vi "Waveform Axis Parameters.vi"(7 "Image Acquisition Parameters":T2={"Scan Type"=enum."Sample Scanning", "Scan Mode"=enum."XY", "Fast Axis Frequency (Hz)"=100.0, "Image Format"=128, "Line Accumulations"=1, "Frames Per Capture"=1, "Frames Accumulations"=1, "Image Dimension (um)"=[], "Number of Z Steps"=1, "Z Steps Size (um)"=1.0, "Pixel Size (nm)"=[], "Customized Image Format"=[]} {"Z Steps Size (um)" min=0.0; "Number of Z Steps" min=1; "Frames Accumulations" min=1; "Frames Per Capture" min=1; "Line Accumulations" min=1; "Image Format" items=["64 x 64"=64, "128 x 128"=128, "256 x 256"=256, "512 x 512"=512, "1024 x 1024"=1024, "2048 x 2048"=2048, "Customized..."=0]}) -> (8 "Scan Parameters":T1)   [LabVIEW 2014]
uses:
  Type Defs/Image Acquisition Parameters.ctl
  Scan Parameters.ctl
panel:
  # "Length"
  # "Height"
  # "XY"
  # "Z"
  # "Length"
  # "Height"
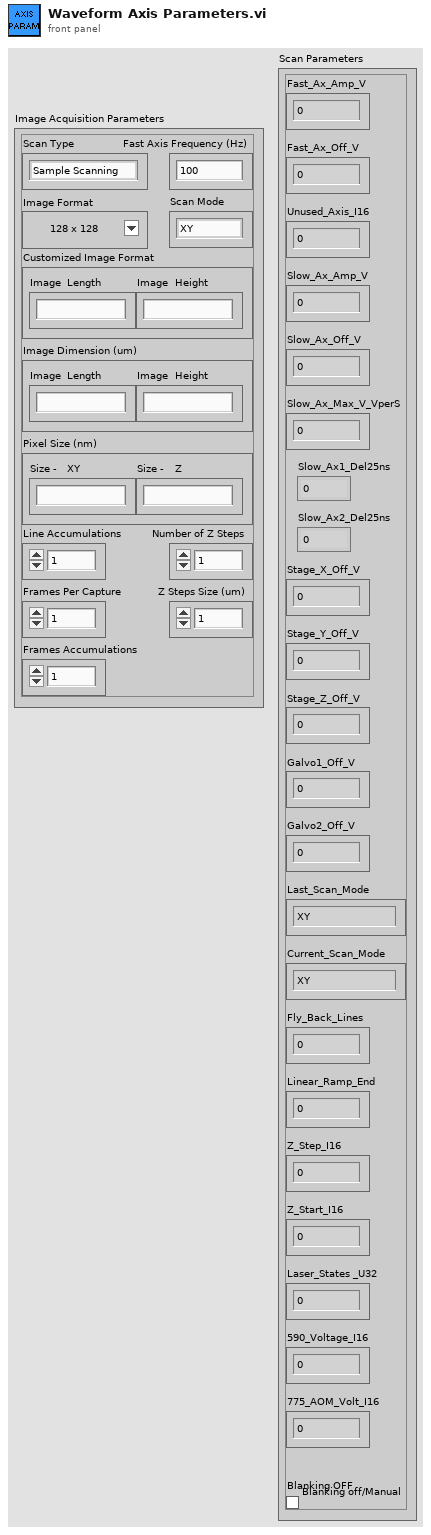
[diagram p1: front panel]
types:
  T1 = typedef "Scan Parameters.ctl" = cluster{"Fast_Ax_Amp_V":dbl, "Fast_Ax_Off_V":dbl, "Slow_Ax_Amp_V":dbl, "Slow_Ax_Off_V ":dbl, "Slow_Ax_Max_V_VperS":dbl, "Slow_Ax1_Del25ns":i32, "Slow_Ax2_Del25ns":i32, "Stage_X_Off_V":dbl, "Stage_Y_Off_V":dbl, "Stage_Z_Off_V":dbl, "Galvo1_Off_V":dbl, "Galvo2_Off_V":dbl, "Last_Scan_Mode":enum16{"XY", "XZ", "YZ", "XYZ"}, "Current_Scan_Mode":enum16{"XY", "XZ", "YZ", "XYZ"}, "Fly_Back_Lines":u16, "Linear_Ramp_End":u32, "Z_Step_I16":i16, "Z_Start_I16":i16, "Laser_States _U32":u32, "590_Voltage_I16":i16, "775_AOM_Volt_I16":i16, "Blanking OFF":bool, "Unused_Axis_I16":i16}
  T2 = typedef "Image Acquisition Parameters.ctl" = cluster{"Scan Type":enum16{"Sample Scanning", "Beam Scanning"}, "Scan Mode":enum16{"XY", "XZ", "YZ", "XYZ"}, "Fast Axis Frequency (Hz)":dbl, "Image Format":u16, "Line Accumulations":u16, "Frames Per Capture":u16, "Frames Accumulations":u16, "Image Dimension (um)":dbl[], "Number of Z Steps":u8, "Z Steps Size (um)":dbl, "Pixel Size (nm)":dbl[], "Customized Image Format":dbl[]}
  T3 = typedef "Scanning Conversions.ctl" = cluster{"Stage X Axis (Volts/um)":dbl, "Stage Y Axis (Volts/um)":dbl, "Stage Z Axis (Volts/um)":dbl}
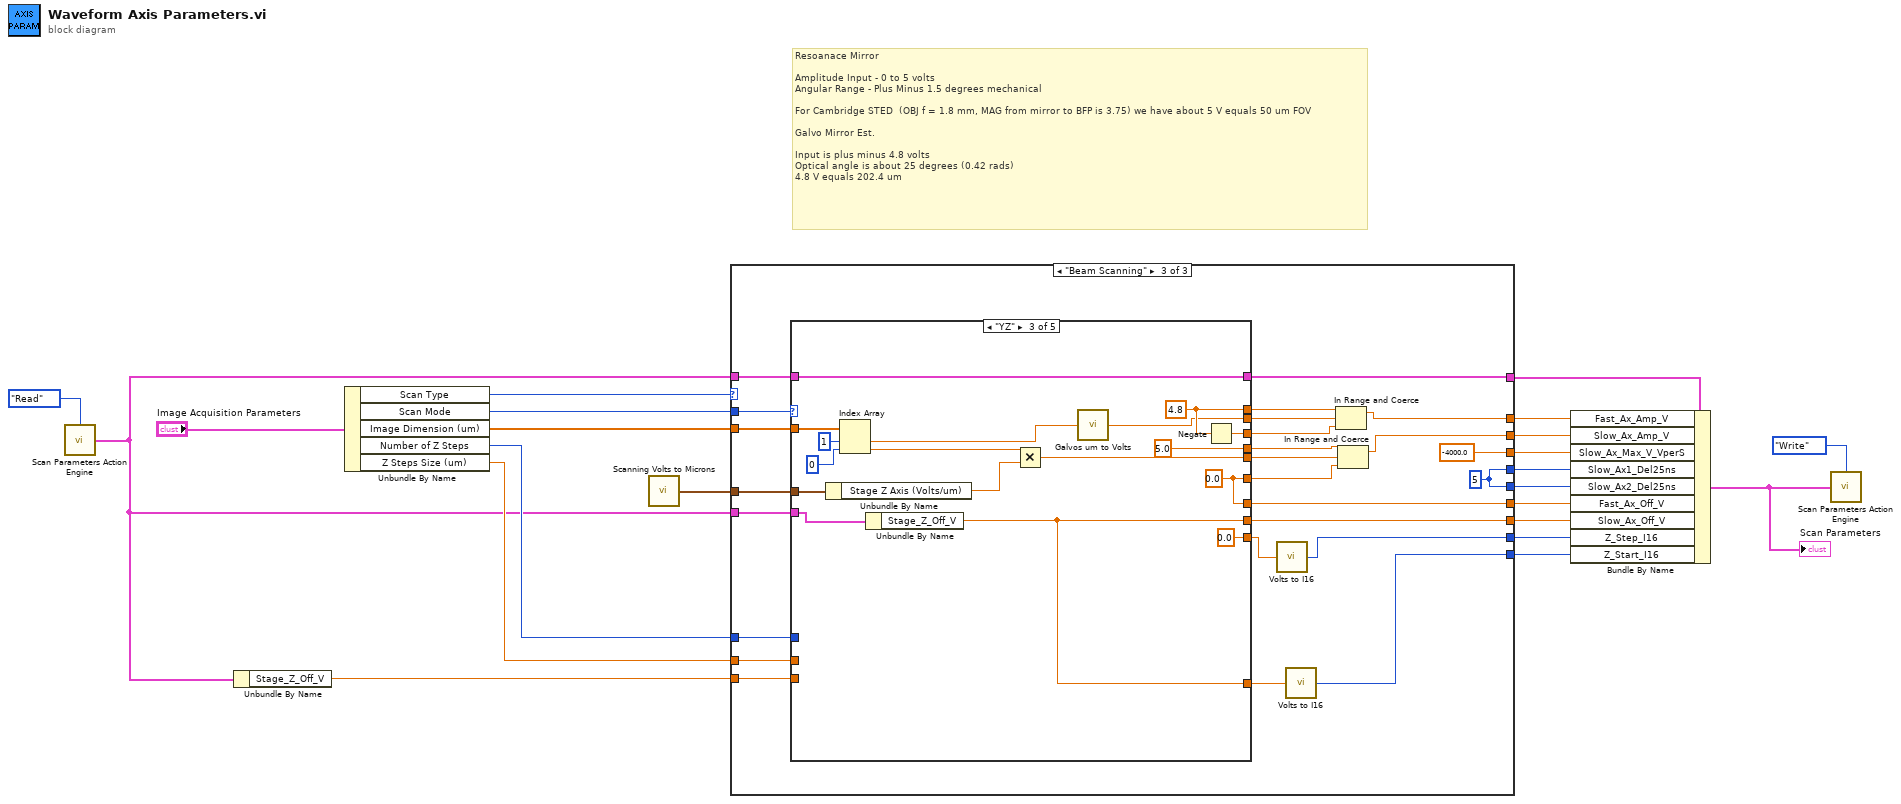
[diagram p0: block diagram]
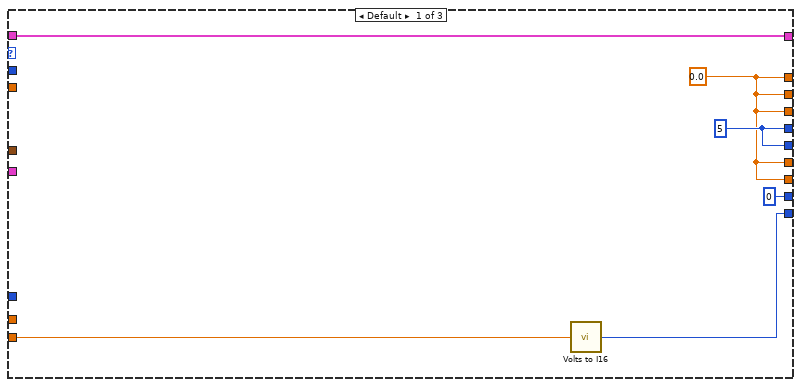
[diagram p2: hidden frame]
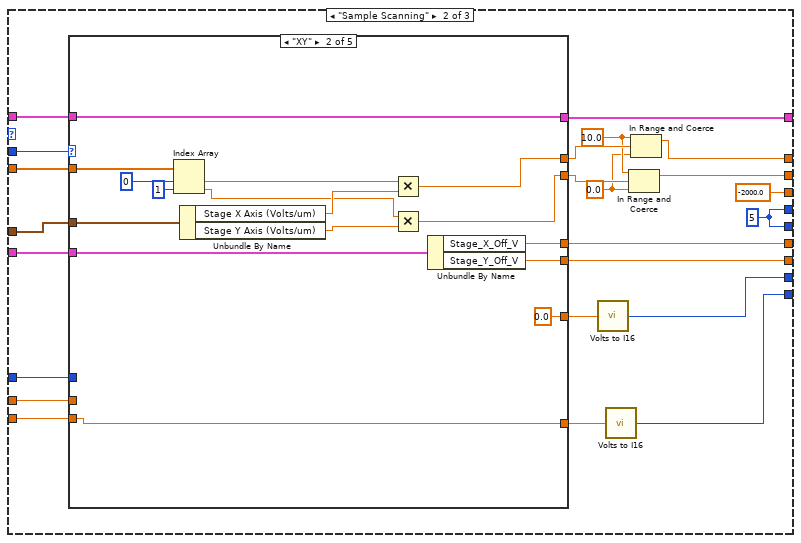
[diagram p3: hidden frame]
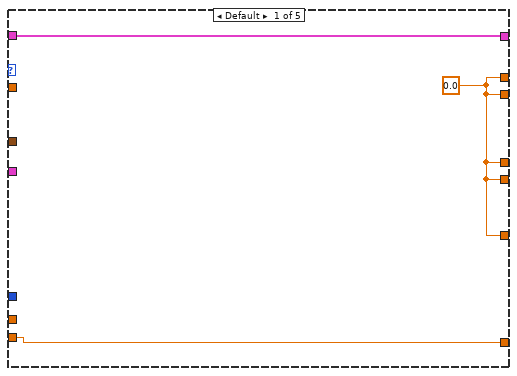
[diagram p4: hidden frame]
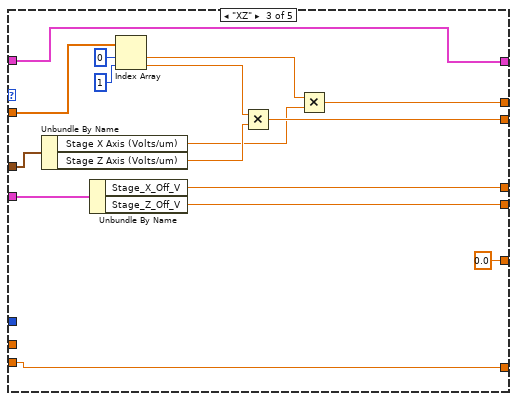
[diagram p5: hidden frame]
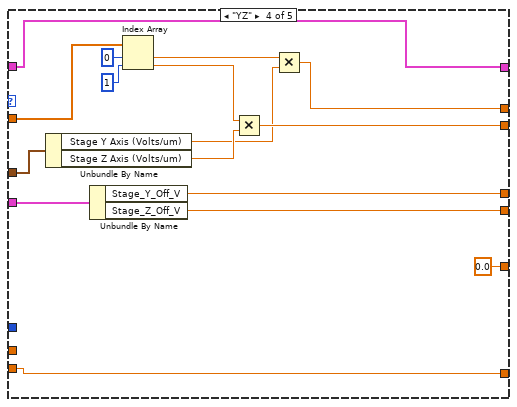
[diagram p6: hidden frame]
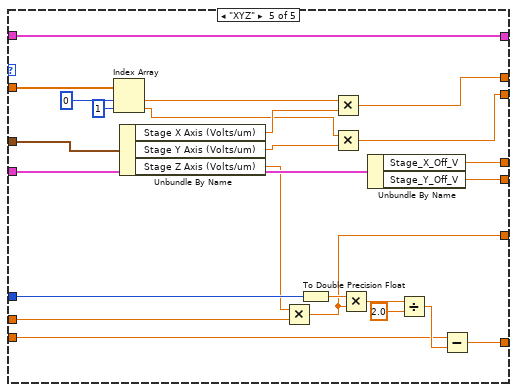
[diagram p7: hidden frame]
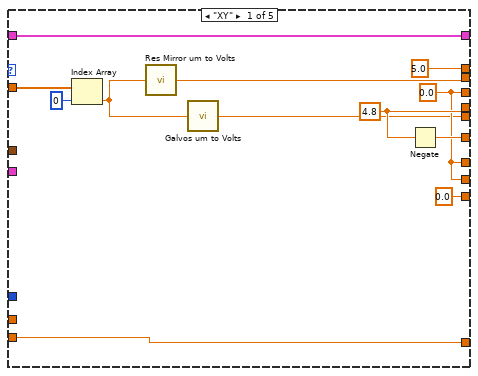
[diagram p8: hidden frame]
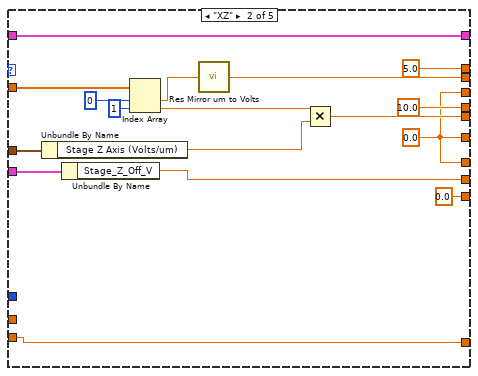
[diagram p9: hidden frame]
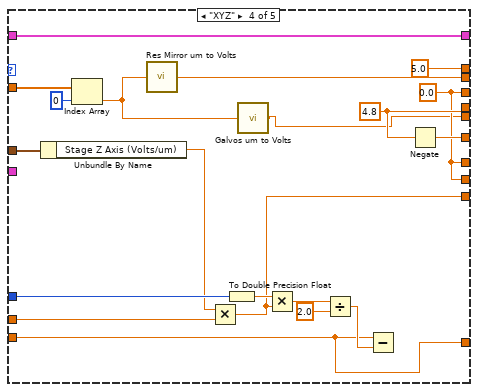
[diagram p10: hidden frame]
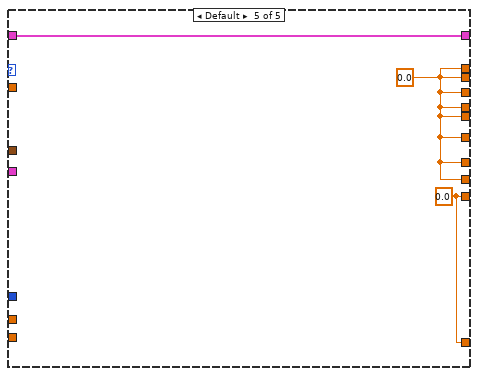
[diagram p11: hidden frame]
diagram:
  # "Resoanace Mirror\n\nAmplitude Input - 0 to 5 volts\nAngular Range - Plus Minus 1.5 degrees mechanical\n\nFor Cambridge STED  (OBJ f = 1.8 mm, MAG from mirror to BFP is 3.75) we have about 5 V equals 50 um FOV\n\nGalvo Mirror Est.\n\nInput is plus minus 4.8 volts\nOptical angle is about 25 degrees (0.42 rads)\n4.8 V equals 202.4 um"
  n1 = call "Scan Parameters Action Engine.vi"("Action"=enum16{"Read", "Write"}."Read") -> ("Scan Parameters OUT"=w4:T1)  [unwired: 14 in]
  n2 = Unbundle By Name(w4) -> ("Stage_Z_Off_V"=w3:dbl)
  n3 = Unbundle By Name("Image Acquisition Parameters") -> ("Scan Type"=w21:enum16{"Sample Scanning", "Beam Scanning"}, "Scan Mode"=w20:enum16{"XY", "XZ", "YZ", "XYZ"}, "Image Dimension (um)"=w19:dbl[], "Number of Z Steps"=w5:u8, "Z Steps Size (um)"=w6:dbl)
  n4 = call "Scanning Volts to Microns.vi"() -> ("Scanning Conversions OUT"=w7:T3)
  n5 = case shown="\"Beam Scanning\"" w21 {
    tunnel: w20 -> [_ w51 w151]
    tunnel: w19 -> [_ w50 w150]
    tunnel: [w27 w38 w141] -> w17
    tunnel: [w27 w37 w142] -> w16
    tunnel: [w27 -2000.0 ("y") -4000.0 ("y")] -> w15
    tunnel: [w28 w48 w148] -> w14
    tunnel: [w28 w48 w148] -> w13
    tunnel: w4 -> [_ w47 w147]
    tunnel: w4 -> [w26 w46 w146]
    tunnel: [w26 w45 w145] -> w9
    tunnel: [w27 w44 w135] -> w12
    tunnel: [w27 w43 w136] -> w11
    tunnel: w7 -> [_ w36 w134]
    tunnel: w6 -> [_ w34 w133]
    tunnel: w5 -> [_ w33 w132]
    tunnel: w3 -> [w25 w35 w131]
    tunnel: [w24 w31 w129] -> w2
    tunnel: [i16 0 ("I16") w29 w127] -> w1
    frame Default {
      w28 = 5 ("Slow Axis 1 Delay (25 ns) Steps")
      w27 = 0.0
      n6 = call "Volts to I16.vi"("Voltage (V)"=w25) -> ("I16"=w24:i16)  [unwired: 13 in, 1 out]
    }
    frame "Sample Scanning" {
      w39 = 0.0 ("lower limit")
      w40 = 10.0 ("upper limit")
      w48 = 5 ("Slow Axis 1 Delay (25 ns) Steps")
      n7 = case shown="\"XY\"" w51 {
        tunnel: w50 -> [_ w69 w86 w98 w125]
        tunnel: [w52 w70 w83 w97 w126] -> w42
        tunnel: [w52 w57 w80 w96 w113] -> w41
        tunnel: w47 -> [_ w66 w78 w94 w122]
        tunnel: w46 -> [w54 w65 w79 w95 w121]
        tunnel: [w54 w65 w79 w95 w121] -> w45
        tunnel: [w52 w64 w77 w93 w120] -> w44
        tunnel: [w52 w63 w76 w92 w119] -> w43
        tunnel: w36 -> [_ w62 w73 w91 w118]
        tunnel: w35 -> [w53 w56 w71 w88 w108]
        tunnel: w34 -> [_ _ _ _ w107]
        tunnel: w33 -> [_ _ _ _ w106]
        tunnel: [w53 w56 w71 w88 w104] -> w32
        tunnel: [w52 0.0 0.0 0.0 w103] -> w30
        frame Default {
          w52 = 0.0
        }
        frame "XY" {
          n8 = Index Array(array=w69, index #1=0 ("index"), index #2=1 ("index")) -> (element #1=w67:dbl, element #2=w59:dbl)
          n9 = Unbundle By Name(w62) -> ("Stage X Axis (Volts/um)"=w60:dbl, "Stage Y Axis (Volts/um)"=w58:dbl)
          n10 = Multiply(x=w67, y=w60) -> (x*y=w70:dbl)
          n11 = Multiply(x=w59, y=w58) -> (x*y=w57:dbl)
          n12 = Unbundle By Name(w66) -> ("Stage_X_Off_V"=w64:dbl, "Stage_Y_Off_V"=w63:dbl)
        }
        frame "XZ" {
          n13 = Unbundle By Name(w73) -> ("Stage X Axis (Volts/um)"=w74:dbl, "Stage Z Axis (Volts/um)"=w75:dbl)
          n14 = Unbundle By Name(w78) -> ("Stage_X_Off_V"=w77:dbl, "Stage_Z_Off_V"=w76:dbl)
          n15 = Index Array(array=w86, index #1=0 ("index"), index #2=1 ("index")) -> (element #1=w84:dbl, element #2=w81:dbl)
          n16 = Multiply(x=w81, y=w75) -> (x*y=w80:dbl)
          n17 = Multiply(x=w84, y=w74) -> (x*y=w83:dbl)
        }
        frame "YZ" {
          n18 = Unbundle By Name(w91) -> ("Stage Y Axis (Volts/um)"=w89:dbl, "Stage Z Axis (Volts/um)"=w90:dbl)
          n19 = Unbundle By Name(w94) -> ("Stage_Y_Off_V"=w93:dbl, "Stage_Z_Off_V"=w92:dbl)
          n20 = Index Array(array=w98, index #1=0 ("index"), index #2=1 ("index")) -> (element #1=w101:dbl, element #2=w99:dbl)
          n21 = Multiply(x=w99, y=w90) -> (x*y=w96:dbl)
          n22 = Multiply(x=w101, y=w89) -> (x*y=w97:dbl)
        }
        frame "XYZ" {
          n23 = Index Array(array=w125, index #1=0 ("index"), index #2=1 ("index")) -> (element #1=w123:dbl, element #2=w115:dbl)
          n24 = Unbundle By Name(w118) -> ("Stage X Axis (Volts/um)"=w116:dbl, "Stage Y Axis (Volts/um)"=w114:dbl, "Stage Z Axis (Volts/um)"=w105:dbl)
          n25 = Multiply(x=w105, y=w107) -> (x*y=w103:dbl)
          n26 = To Double Precision Float(number=w106) -> (double precision float=w112:dbl)
          n27 = Multiply(x=w123, y=w116) -> (x*y=w126:dbl)
          n28 = Multiply(x=w115, y=w114) -> (x*y=w113:dbl)
          n29 = Multiply(x=w112, y=w103) -> (x*y=w111:dbl)
          n30 = Unbundle By Name(w122) -> ("Stage_X_Off_V"=w120:dbl, "Stage_Y_Off_V"=w119:dbl)
          n31 = Divide(x=w111, y=2.0) -> (x/y=w109:dbl)
          n32 = Subtract(x=w108, y=w109) -> (x-y=w104:dbl)
        }
      }
      n33 = call "Volts to I16.vi"("Voltage (V)"=w30) -> ("I16"=w29:i16)  [unwired: 13 in, 1 out]
      n34 = call "Volts to I16.vi"("Voltage (V)"=w32) -> ("I16"=w31:i16)  [unwired: 13 in, 1 out]
      n35 = In Range and Coerce(upper limit=w40, x=w41, lower limit=w39) -> (coerced(x)=w37:dbl)  [unwired: 1 out]
      n36 = In Range and Coerce(upper limit=w40, x=w42, lower limit=w39) -> (coerced(x)=w38:dbl)  [unwired: 1 out]
    }
    frame "Beam Scanning" {
      w148 = 5 ("Slow Axis 1 Delay (25 ns) Steps")
      n37 = case shown="\"YZ\"" w151 {
        tunnel: w150 -> [w162 w179 w195 w216 _]
        tunnel: w147 -> [_ w175 w190 _ _]
        tunnel: [w163 w172 w197 w217 w220] -> w145
        tunnel: w146 -> [w163 w172 w197 w217 w220]
        tunnel: [w154 w167 w182 w201 w219] -> w144
        tunnel: [w152 w178 w194 w199 w219] -> w143
        tunnel: [5.0 5.0 w193 5.0 w219] -> w140
        tunnel: [w157 w173 w192 w211 w219] -> w139
        tunnel: [w159 10.0 5.0 w213 w219] -> w138
        tunnel: [w158 w173 w189 w212 w219] -> w137
        tunnel: [w157 w174 w181 w211 w219] -> w136
        tunnel: [w157 w173 w189 w211 w219] -> w135
        tunnel: w134 -> [_ w171 w188 w210 _]
        tunnel: w133 -> [_ _ _ w204 _]
        tunnel: w132 -> [_ _ _ w209 _]
        tunnel: w131 -> [w155 w168 _ w198 _]
        tunnel: [w155 w168 w181 w198 w218] -> w130
        tunnel: [0.0 ("I16") 0.0 ("I16") 0.0 ("I16") w202 w218] -> w128
        frame "XY" {
          w159 = 4.8
          w157 = 0.0
          n38 = Index Array(array=w162, index=0) -> (element=w153:dbl)
          n39 = call "Res Mirror um to Volts.vi"("Image Size (um)"=w153) -> ("Voltage (V)"=w154:dbl)
          n40 = call "Galvos um to Volts.vi"("Image Size (um)"=w153) -> ("Voltage (V)"=w152:dbl)
          n41 = Negate(x=w159) -> (-x=w158:dbl)
        }
        frame "XZ" {
          w173 = 0.0
          n42 = Unbundle By Name(w171) -> ("Stage Z Axis (Volts/um)"=w170:dbl)
          n43 = Unbundle By Name(w175) -> ("Stage_Z_Off_V"=w174:dbl)
          n44 = Index Array(array=w179, index #1=0 ("index"), index #2=1 ("index")) -> (element #1=w166:dbl, element #2=w164:dbl)
          n45 = call "Res Mirror um to Volts.vi"("Image Size (um)"=w166) -> ("Voltage (V)"=w167:dbl)
          n46 = Multiply(x=w164, y=w170) -> (x*y=w178:dbl)
        }
        frame "YZ" {
          w189 = 0.0
          w193 = 4.8
          n47 = Unbundle By Name(w188) -> ("Stage Z Axis (Volts/um)"=w187:dbl)
          n48 = Index Array(array=w195, index #1=1 ("index"), index #2=0 ("index")) -> (element #1=w183:dbl, element #2=w184:dbl)
          n49 = Unbundle By Name(w190) -> ("Stage_Z_Off_V"=w181:dbl)
          n50 = Multiply(x=w184, y=w187) -> (x*y=w194:dbl)
          n51 = call "Galvos um to Volts.vi"("Image Size (um)"=w183) -> ("Voltage (V)"=w182:dbl)
          n52 = Negate(x=w193) -> (-x=w192:dbl)
        }
        frame "XYZ" {
          w213 = 4.8
          w211 = 0.0
          n53 = Unbundle By Name(w210) -> ("Stage Z Axis (Volts/um)"=w203:dbl)
          n54 = Index Array(array=w216, index=0) -> (element=w200:dbl)
          n55 = call "Res Mirror um to Volts.vi"("Image Size (um)"=w200) -> ("Voltage (V)"=w201:dbl)
          n56 = Multiply(x=w203, y=w204) -> (x*y=w202:dbl)
          n57 = To Double Precision Float(number=w209) -> (double precision float=w208:dbl)
          n58 = call "Galvos um to Volts.vi"("Image Size (um)"=w200) -> ("Voltage (V)"=w199:dbl)
          n59 = Multiply(x=w208, y=w202) -> (x*y=w207:dbl)
          n60 = Divide(x=w207, y=2.0) -> (x/y=w205:dbl)
          n61 = Subtract(x=w198, y=w205) -> ()  [unwired: 1 out]
          n62 = Negate(x=w213) -> (-x=w212:dbl)
        }
        frame Default {
          w218 = 0.0 ("I16")
          w219 = 0.0
        }
      }
      n63 = call "Volts to I16.vi"("Voltage (V)"=w128) -> ("I16"=w127:i16)  [unwired: 13 in, 1 out]
      n64 = call "Volts to I16.vi"("Voltage (V)"=w130) -> ("I16"=w129:i16)  [unwired: 13 in, 1 out]
      n65 = In Range and Coerce(upper limit=w140, x=w144, lower limit=w139) -> (coerced(x)=w141:dbl)  [unwired: 1 out]
      n66 = In Range and Coerce(upper limit=w138, x=w143, lower limit=w137) -> (coerced(x)=w142:dbl)  [unwired: 1 out]
    }
  }
  n67 = Bundle By Name(cluster=w9, "Fast_Ax_Amp_V"=w17, "Slow_Ax_Amp_V"=w16, "Slow_Ax_Max_V_VperS"=w15, "Slow_Ax1_Del25ns"=w14, "Slow_Ax2_Del25ns"=w13, "Fast_Ax_Off_V"=w12, "Slow_Ax_Off_V"=w11, "Z_Step_I16"=w1, "Z_Start_I16"=w2) -> (w8:T1)
  "Scan Parameters" <- w8
  n68 = call "Scan Parameters Action Engine.vi"("Action"=enum16{"Read", "Write"}."Write", "Scan Parameters IN"=w8) -> ()  [unwired: 13 in, 1 out]
